vi "Msg Receive.vi"(11 "Process in":refnum<class "Process.lvclass">) -> (0 "error out":errorcluster, 1 "Destroyed Self?":bool, 3 "Process out":refnum<class "Process.lvclass">)   [LabVIEW 2021, in "Process.lvlib" / "Process.lvclass"]
uses:
  Process.lvclass
  Process.lvclass/Process.ctl
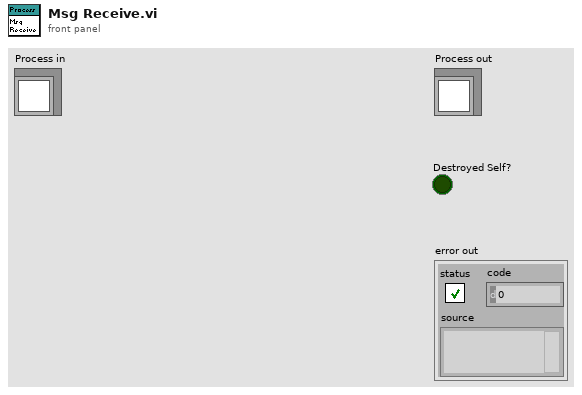
[diagram p1: front panel]
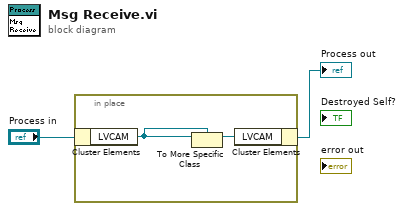
[diagram p0: block diagram]
diagram:
  n1 = in-place {
    n2 = in-place-cluster #1("Process in") -> ("LVCAM"=w3:refnum<class "LVCAM.lvclass">)
    n3 = To More Specific Class(target class=w3, reference=w3) -> (specific class reference=w4:refnum<class "LVCAM.lvclass">)  [unwired: 1 in, 1 out]
    n4 = in-place-cluster #1("LVCAM"=w4) -> (→"Process out":refnum<class "Process.lvclass">)
  }
